vi "Power Clear Request.vi"(8 "error in (no error)":errorcluster, 10 "Power Request Type":T1, 11 "Handle in":i64) -> (0 "error out":errorcluster, 2 "Success?":bool, 3 "Handle out":i64)   [LabVIEW 2024, in "Request Power.lvlib"]
uses:
  Request Power.lvlib
  typedefs/Power Request Type.ctl
  kernel32.dll
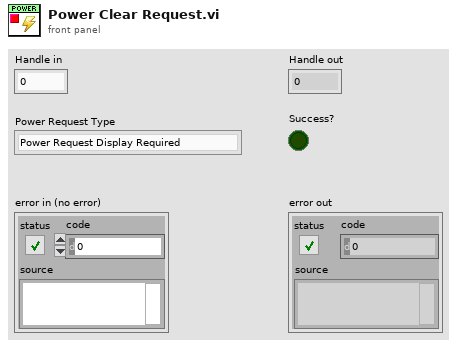
[diagram p1: front panel]
types:
  T1 = typedef "Request Power.lvlib/Power Request Type.ctl" = enum32{"Power Request Display Required", "Power Request System Required", "Power Request Away Mode Required", "Power Request Execution Required"}
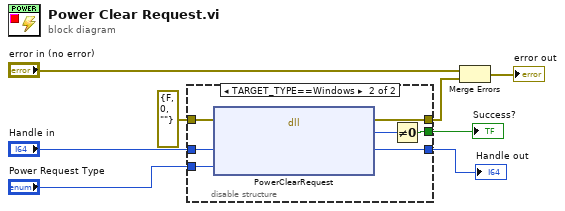
[diagram p0: block diagram]
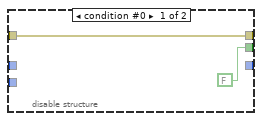
[diagram p2: hidden frame]
diagram:
  n1 = disable-structure shown="TARGET_TYPE==Windows" {
    disable-tunnel: [w10 w17] -> w4
    disable-tunnel: errorcluster {"status"=FALSE, "code"=0, "source"=""} ("error in (no error)") -> [w10 w16]
    disable-tunnel: "Handle in" -> [_ w15]
    disable-tunnel: "Power Request Type" -> [_ w14]
    disable-tunnel: [FALSE w12] -> w6
    disable-tunnel: [_ w11] -> w1
    frame condition #0 {
    }
    frame condition #1 (active) {
      n2 = dll-call lib="kernel32.dll" fn="PowerClearRequest"(error in=w16, "_In_ HANDLE"=w15, "_In_ POWER_REQUEST_TYPE"=w14) -> (error out=w17:errorcluster, "BOOL"=w13:i32, "_In_ HANDLE"=w11:i64)  [unwired: 3 in, 1 out]
      n3 = Not Equal To 0?(x=w13) -> (x != 0?=w12:bool)
    }
  }
  "Success?" <- w6
  "Handle out" <- w1
  n4 = Merge Errors("error in (no error)", w4) -> (→"error out":errorcluster)
